vi "CLSUIP_CreateNewVI.vi"(0 "VIRetooler":refnum<class "VIRetooler.lvclass">, 3 "error in (no error)":errorcluster) -> (6 "VIRetooler out":refnum<class "VIRetooler.lvclass">, 9 "error out":errorcluster)   [LabVIEW 2021, in "MemberVICreation.lvlib" / "VIRetooler.lvclass"]
uses:
  <resource>/Framework/Providers/LVClassLibrary/NewAccessors/VIRetooler/VIRetooler.lvclass
  <resource>/Framework/Providers/LVClassLibrary/NewAccessors/VIRetooler/VIRetooler.lvclass/VIRetooler.ctl
  <resource>/Framework/Providers/LVClassLibrary/NewAccessors/MemberVICreation.lvlib
panel:
  out "Block Diagram":refnum<vi>
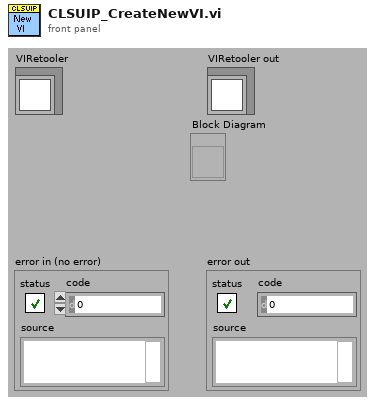
[diagram p1: front panel]
types:
  T1 = typedef "imagedata.ctl" = cluster{"image type":i32, "image depth":i32, "image":u8[], "mask":u8[], "colors":u32[], "Rectangle":cluster{"left":i16, "top":i16, "right":i16, "bottom":i16}}
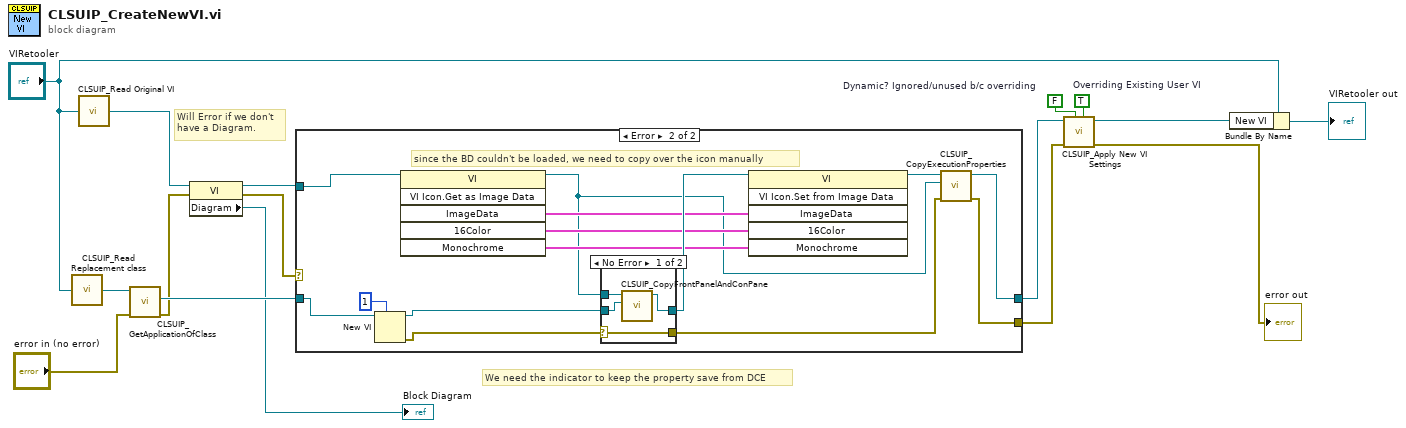
[diagram p0: block diagram]
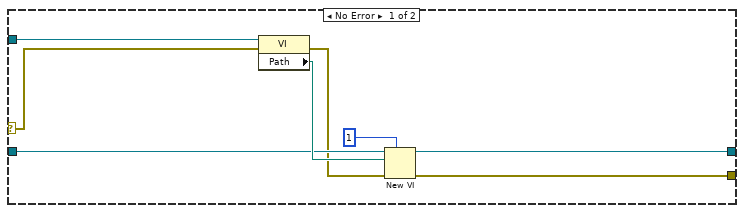
[diagram p2: hidden frame]
diagram:
  w1 = FALSE  # Dynamic? Ignored/unused b/c overriding
  w2 = TRUE  # Overriding Existing User VI
  # "Will Error if we don't\nhave a Diagram."
  # "We need the indicator to keep the property save from DCE"
  n1 = call <resource>:"CLSUIP_Read Replacement class.vi"("VIRetooler.lvclass in"="VIRetooler") -> ("Replacement class"=w16:refnum<vi>)
  n2 = call <resource>:"CLSUIP_Read Original VI.vi"("VIRetooler.lvclass in"="VIRetooler") -> ("Original VI"=w8:refnum<vi>)
  n3 = call <resource>:"CLSUIP_GetApplicationOfClass.vi"("error in (no error)"="error in (no error)", "LVClassLibrary Ref"=w16) -> ("error out"=w7:errorcluster, "Application"=w15:refnum<vi>)  [unwired: 8 out]
  n4 = property class="VI"(reference=w8, error in=w7) -> (reference out=w5:refnum<vi>, error out=w6:errorcluster, "Diagram"=→"Block Diagram":refnum<vi>)
  n5 = case shown="Error" w6 {
    selector: w6 -> [w17 _]
    tunnel: w15 -> [w23 w37]
    tunnel: w5 -> [w20 w34]
    tunnel: [w19 w28] -> w11
    tunnel: [w18 w25] -> w10
    frame No Error {
      n6 = property on="Property Node" class="VI"(reference=w20, error in=w17) -> (error out=w22:errorcluster, "Path"=w24:path)  [unwired: 1 out]
      n7 = New VI(7:u32 1 ("options"), 8:w22, 10:w24, 11:w23) -> (0:w18:errorcluster, 3:w19:refnum<vi>)  [unwired: 1 in, 2 out]
    }
    frame Error {
      # "since the BD couldn't be loaded, we need to copy over the icon manually"
      n8 = New VI(7:u32 1 ("options"), 11:w37) -> (0:w35:errorcluster, 3:w36:refnum<vi>)  [unwired: 3 in, 2 out]
      n9 = invoke class="VI" method="VI Icon.Get as Image Data"(reference=w34) -> (reference out=w27:refnum<vi>, "ImageData"=w32:T1, "16Color"=w31:T1, "Monochrome"=w30:T1)  [unwired: 5 in, 2 out]
      n10 = case shown="No Error" w35 {
        selector: w35 -> [w39 w44]
        tunnel: w36 -> [w42 w43]
        tunnel: w27 -> [w41 _]
        tunnel: [w40 w43] -> w33
        tunnel: [w39 w44] -> w26
        frame No Error {
          n11 = call <resource>:"CLSUIP_CopyFrontPanelAndConPane.vi"("New VI"=w42, "Orig VI"=w41) -> ("New VI out"=w40:refnum<vi>)  [unwired: 9 in]
        }
        frame Error {
        }
      }
      n12 = invoke class="VI" method="VI Icon.Set from Image Data"(reference=w33, "ImageData"=w32, "16Color"=w31, "Monochrome"=w30) -> (reference out=w29:refnum<vi>)  [unwired: 2 in, 5 out]
      n13 = call <resource>:"CLSUIP_CopyExecutionProperties.vi"("error in (no error)"=w26, "Old VI in"=w27, "New VI in"=w29) -> ("error out"=w25:errorcluster, "New VI out"=w28:refnum<vi>)  [unwired: 7 in]
    }
  }
  n14 = call <resource>:"CLSUIP_Apply New VI Settings.vi"("Overriding Existing User VI"=w2, "Making dynamic?"=w1, "error in"=w10, "VI in"=w11) -> ("error out"=→"error out":errorcluster, "VI out"=w12:refnum<vi>)  [unwired: 6 in]
  n15 = Bundle By Name(cluster="VIRetooler", "New VI"=w12) -> (→"VIRetooler out":refnum<class "VIRetooler.lvclass">)
